vi "CreatePrivateEvents.vi"(8 "error in (no error)":errorcluster, 11 "DAQ":refnum<class "DAQ.lvclass">) -> (0 "error out":errorcluster, 3 "DAQ out":refnum<class "DAQ.lvclass">)   [LabVIEW 2016, in "DAQ.lvclass"]
doc: "---------------------------------------------------------------\nJKI State Machine Objects™\nhttp://jki.net/state-machine-objects/\nCopyright (C) 2005-2015, JKI <info@jki.net>\nALL RIGHTS RESERVEDJKI State Machine Objects (SMO) 1.0.0.4\nJKI - JKI\nCopyright (c) 2015, JKI"
uses:
  DAQ.lvclass
  Typedefs/PrivateEvents--DAQ.AI.Channels.ctl
  Typedefs/PrivateEvents--DAQ.AO.Channels.ctl
  Typedefs/PrivateEvents--DAQ.Write.ctl
  DAQ.lvclass/DAQ.ctl
  <vilib>/JKI/JKI SMO/SMO/SMO.lvclass
panel:
  # "For instructions on how to use the JKI State Machine Objects, examples and video tutorials, visit:\nhttp://jki.net/state-machine-objects/\n\nJKI State Machine Objects™\nhttp://jki.net/state-machine-objects/\nCopyright (C) 2005-2015, JKI <info@jki.net>\nALL RIGHTS RESERVED"
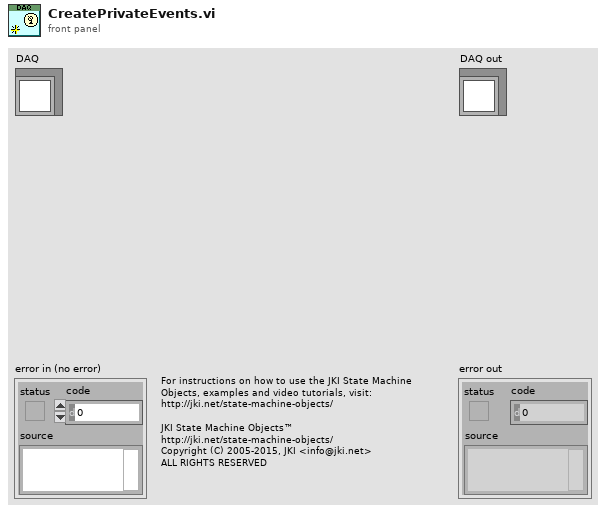
[diagram p1: front panel]
types:
  T1 = typedef "DAQ.lvclass/PrivateEvents--DAQ.Write.ctl" = waveform(dbl)[]
  T2 = typedef "DAQ.lvclass/PrivateEvents--DAQ.AO.Channels.ctl" = string
  T3 = typedef "DAQ.lvclass/PrivateEvents--DAQ.AI.Channels.ctl" = string
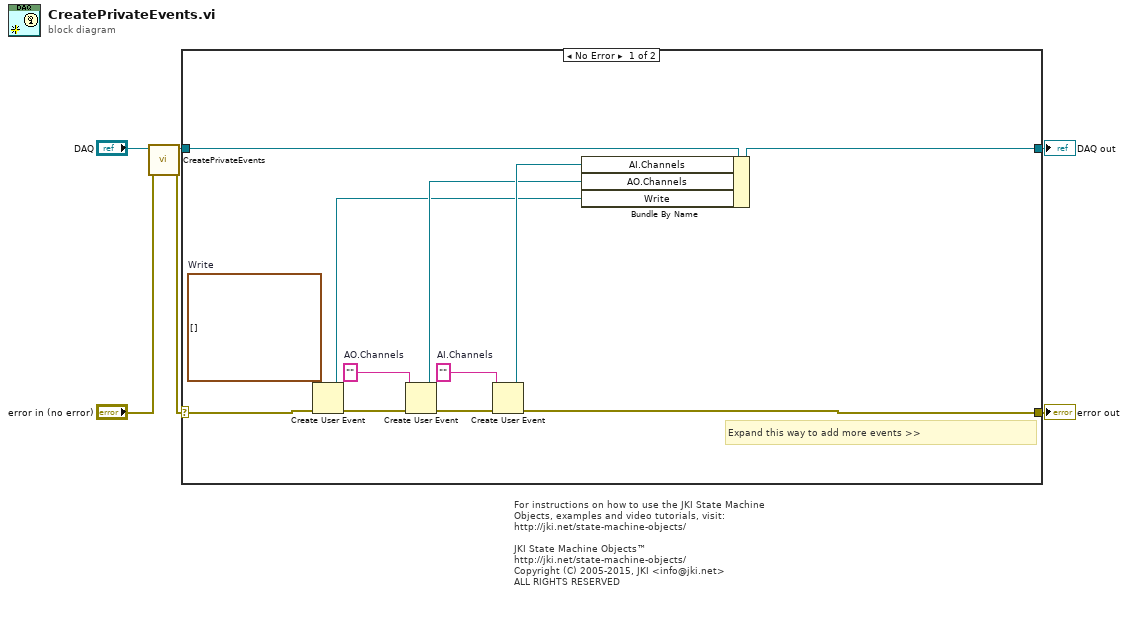
[diagram p0: block diagram]
diagram:
  # "For instructions on how to use the JKI State Machine Objects, examples and video tutorials, visit:\nhttp://jki.net/state-machine-objects/\n\nJKI State Machine Objects™\nhttp://jki.net/state-machine-objects/\nCopyright (C) 2005-2015, JKI <info@jki.net>\nALL RIGHTS RESERVED"
  n1 = call-parent "CreatePrivateEvents.vi"("error in (no error)"="error in (no error)", "SMO"="DAQ") -> ("error out"=w1:errorcluster, "SMO out"=w3:refnum<class "DAQ.lvclass">)  [unwired: 8 in]
  n2 = case shown="No Error" w1 {
    selector: w1 -> [w17 w20]
    tunnel: [w15 w20] -> w5
    tunnel: [w16 w19] -> w6
    tunnel: w3 -> [w18 w19]
    frame No Error {
      w8 = T1 []  # Write
      w11 = T2 ""  # AO.Channels
      w14 = T3 ""  # AI.Channels
      # "Expand this way to add more events >>"
      n3 = Create User Event(user event datatype=w8, error in=w17) -> (user event=w7:refnum<user-event>, error out=w9:errorcluster)
      n4 = Create User Event(user event datatype=w11, error in=w9) -> (user event=w10:refnum<user-event>, error out=w12:errorcluster)
      n5 = Create User Event(user event datatype=w14, error in=w12) -> (user event=w13:refnum<user-event>, error out=w15:errorcluster)
      n6 = Bundle By Name(cluster=w18, "AI.Channels"=w13, "AO.Channels"=w10, "Write"=w7) -> (w16:refnum<class "DAQ.lvclass">)
    }
    frame Error {
    }
  }
  "error out" <- w5
  "DAQ out" <- w6
